vi "Handle HTTP Error Reply.vi"(7 "Bad Request (F)":bool, 8 "error in (no error)":errorcluster, 9 "Additional HTTP Log data":string[](array[string]), 10 "HTTP Status Code":T1={"HTTP Code"=200, "JSON Response"={"error"="No Error", "reason"="No Error"}}, 11 "Web Request in":refnum<class "Web Request.lvclass">) -> (3 "Web Request out":refnum<class "Web Request.lvclass">)   [LabVIEW 2016, in "WSsupport.lvlib"]
uses:
  WSsupport.lvlib
  <vilib>/wsapi/Web Request.lvclass
  ServerErrors/Error Message--cluster.ctl
  <vilib>/Utility/error.llb/DialogType.ctl
  ServerErrors/ServerErrors.lvlib
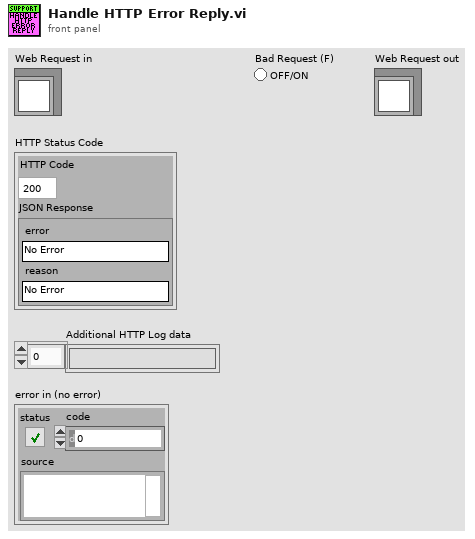
[diagram p1: front panel]
types:
  T1 = typedef "ServerErrors.lvlib/Error Message--cluster.ctl" = cluster{"HTTP Code":i32, "JSON Response":cluster{"error":string, "reason":string}}
  T2 = typedef "DialogType.ctl" = u16
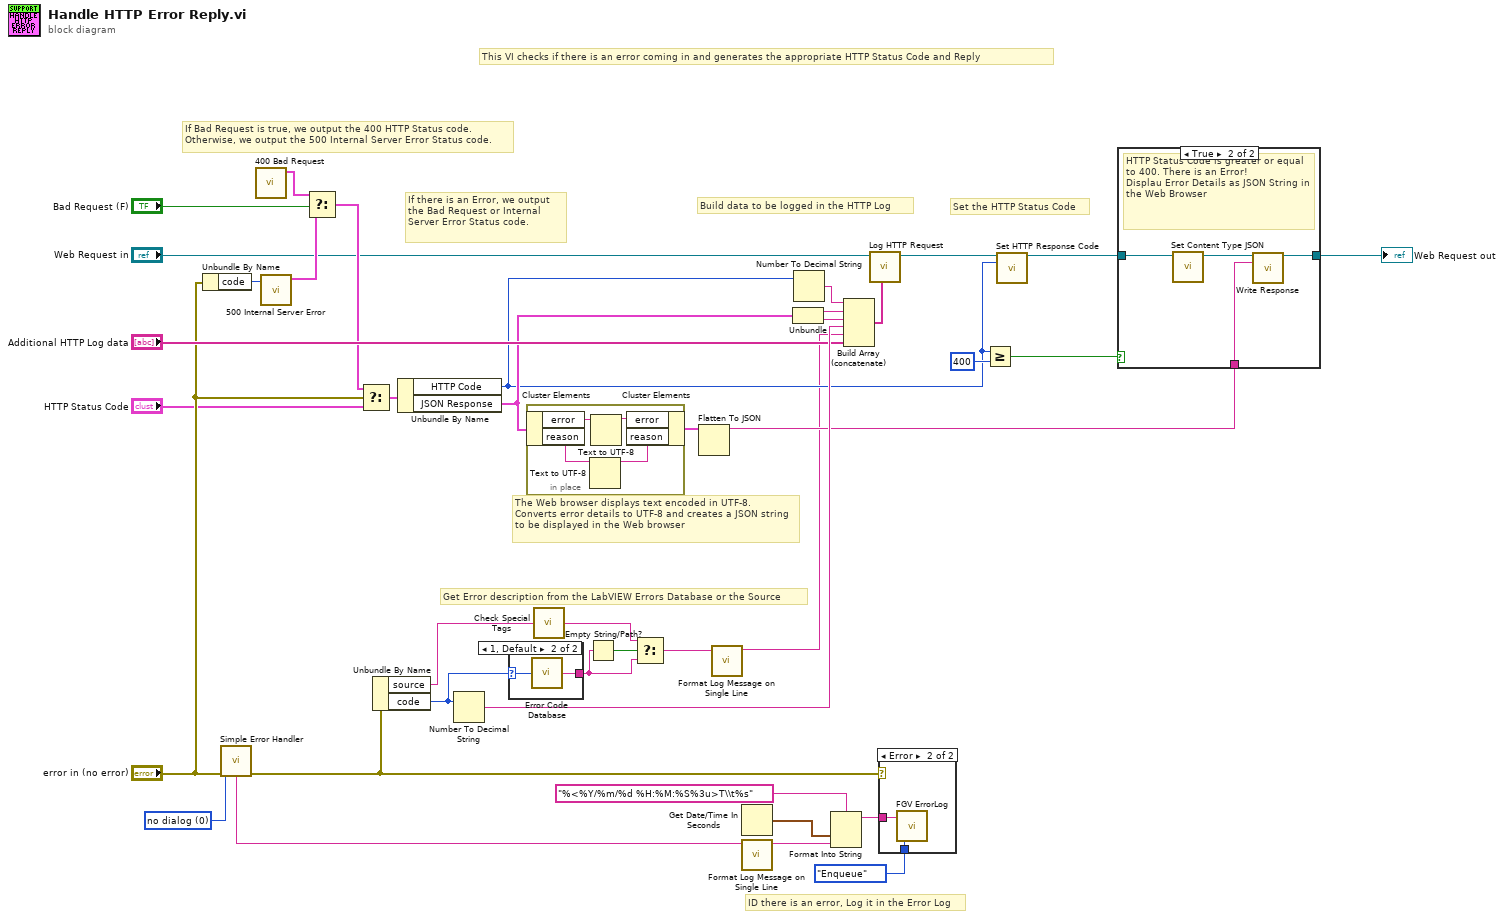
[diagram p0: block diagram]
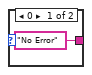
[diagram p3: hidden frame]
diagram:
  w39 = T2 0 items=["no dialog", "OK message", "continue or stop message", "OK message + warnings", "continue/stop + warnings"] ("type of dialog (OK msg:1)")
  # "Set the HTTP Status Code"
  # "Get Error description from the LabVIEW Errors Database or the Source"
  # "The Web browser displays text encoded in UTF-8.\nConverts error details to UTF-8 and creates a JSON string to be displayed in the Web browser"
  # "ID there is an error, Log it in the Error Log"
  # "Build data to be logged in the HTTP Log"
  # "This VI checks if there is an error coming in and generates the appropriate HTTP Status Code and Reply"
  # "If there is an Error, we output the Bad Request or Internal Server Error Status code."
  # "If Bad Request is true, we output the 400 HTTP Status code.\nOtherwise, we output the 500 Internal Server Error Status code."
  n1 = Unbundle By Name("error in (no error)") -> ("code"=w22:i32)
  n2 = call <vilib>:"Simple Error Handler.vi"("type of dialog (OK msg:1)"=w39, "error in (no error)"="error in (no error)") -> ("error out"=w32:errorcluster, "message"=w38:string)  [unwired: 3 in, 3 out]
  n3 = call "400 Bad Request.vi"() -> ("error"=w5:T1)  [unwired: 11 in]
  n4 = call "500 Internal Server Error.vi"("LabVIEW Error Code"=w22) -> ("Error"=w7:T1)  [unwired: 10 in]
  n5 = Select(t=w5, s="Bad Request (F)", f=w7) -> (s? t:f=w8:T1)
  n6 = Select(t=w8, s="error in (no error)", f="HTTP Status Code") -> (s? t:f=w21:T1)
  n7 = Unbundle By Name(w32) -> ("source"=w31:string, "code"=w33:i32)
  n8 = Unbundle By Name(w21) -> ("HTTP Code"=w9:i32, "JSON Response"=w19:cluster{"error":string, "reason":string})
  n9 = Number To Decimal String(number=w33) -> (decimal integer string=w27:string)  [unwired: 1 in]
  n10 = case shown="1, Default" w33 {
    selector: w33 -> [_ w41]
    tunnel: ["No Error" ("Error Text") w42] -> w28
    frame 0 {
    }
    frame 1, Default {
      n11 = call <vilib>:"Error Code Database.vi"("Error Code"=w41) -> ("Error Text"=w42:string)
    }
  }
  n12 = in-place {
    n13 = in-place-cluster #1(w19) -> ("error"=w44:string, "reason"=w46:string)
    n14 = Text to UTF-8(11:w46) -> (3:w45:string)  [unwired: 2 in, 1 out]
    n15 = Text to UTF-8(11:w44) -> (3:w43:string)  [unwired: 2 in, 1 out]
    n16 = in-place-cluster #1("error"=w43, "reason"=w45) -> (w16:cluster{"error":string, "reason":string})
  }
  n17 = call <vilib>:"Check Special Tags.vi"("source"=w31) -> ("After Tag (special data)"=w29:string)  [unwired: 2 out]
  n18 = Empty String/Path?(string/path=w28) -> (empty?=w30:bool)
  n19 = Select(t=w29, s=w30, f=w28) -> (s? t:f=w2:string)
  n20 = Flatten To JSON(anything=w16) -> (JSON string=w14:string)  [unwired: 2 in, 1 out]
  n21 = call "Format Log Message on Single Line.vi"("Log Message"=w2) -> ("Formatted Log Message"=w1:string)  [unwired: 10 in]
  n22 = Get Date/Time In Seconds() -> (seconds since 1Jan1904=w36:timestamp)
  n23 = call "Format Log Message on Single Line.vi"("Log Message"=w38) -> ("Formatted Log Message"=w4:string)  [unwired: 10 in]
  n24 = Unbundle(w19) -> ("error"=w18:string, "reason"=w17:string)
  n25 = Number To Decimal String(number=w9) -> (decimal integer string=w11:string)  [unwired: 1 in]
  n26 = Format Into String(format string="%<%Y/%m/%d %H:%M:%S%3u>T\\t%s", w36, w4) -> (resulting string=w35:string)  [unwired: 2 in, 1 out]
  n27 = Build Array (concatenate)(w11, w18, w17, w27, w1, "Additional HTTP Log data") -> (w25:string[])
  n28 = call "Log HTTP Request.vi"("Error information"=w25, "LabVIEW Web Service Request"="Web Request in") -> ("LabVIEW Web Service Request out"=w26:refnum<class "Web Request.lvclass">)  [unwired: 8 in, 1 out]
  n29 = case shown="Error" w32 {
    tunnel: w35 -> [_ w48]
    tunnel: enum16{"Reset", "Enqueue", "Dequeue"}."Enqueue" ("Action") -> [_ w47]
    frame No Error {
    }
    frame Error {
      n30 = call "FGV ErrorLog.vi"("Action"=w47, "String to log"=w48) -> ()  [unwired: 1 in, 1 out]
    }
  }
  n31 = Greater Or Equal?(x=w9, y=400) -> (x >= y?=w13:bool)
  n32 = call <vilib>:"Set HTTP Response Code.vi"("LabVIEW Web Service Request"=w26, "response code (200)"=w9) -> ("LabVIEW Web Service Request out"=w10:refnum<class "Web Request.lvclass">)  [unwired: 12 in, 1 out]
  n33 = case shown="True" w13 {
    tunnel: w10 -> [w49 w53]
    tunnel: [w49 w52] -> w15
    tunnel: w14 -> [_ w51]
    frame False {
      # "HTTP Status Code is less than 400. No Error"
    }
    frame True {
      # "HTTP Status Code is greater or equal to 400. There is an Error!\nDisplau Error Details as JSON String in the Web Browser"
      n34 = call "Set Content Type JSON.vi"("LabVIEW Web Service Request"=w53) -> ("LabVIEW Web Service Request out"=w50:refnum<class "Web Request.lvclass">)  [unwired: 9 in, 1 out]
      n35 = call <vilib>:"Write Response.vi"("LabVIEW Web Service Request"=w50, "response string"=w51) -> ("LabVIEW Web Service Request out"=w52:refnum<class "Web Request.lvclass">)  [unwired: 12 in, 1 out]
    }
  }
  "Web Request out" <- w15
